vi "Obtain Message Queue.vi"(8 "error in (no error)":errorcluster) -> (0 "error out":errorcluster, 3 "Message Queue":refnum<queue>)   [LabVIEW 2020, in "Polar Bear Plus All-in-One Plugin.lvlib" / "Message Queue.lvlib"]
doc: "Create a queue with the Message Cluster data type."
uses:
  Message Queue.lvlib
  Message Cluster.ctl
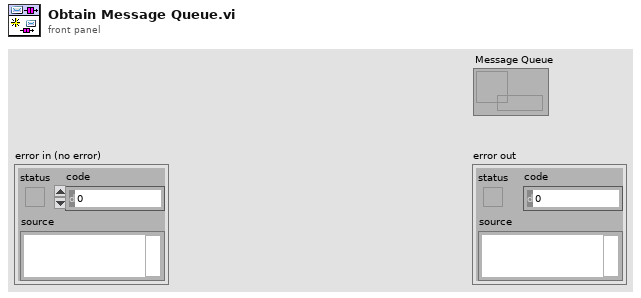
[diagram p1: front panel]
types:
  T1 = typedef "Polar Bear Plus All-in-One Plugin.lvlib/Message Queue.lvlib/Message Cluster.ctl" = cluster{"Message":string, "Message Data":variant}
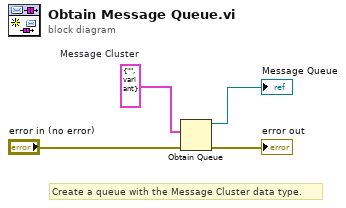
[diagram p0: block diagram]
diagram:
  w4 = T1 {"Message"="", "Message Data"=variant}  # Message Cluster
  # "Create a queue with the Message Cluster data type."
  n1 = Obtain Queue(element data type=w4, error in (no error)="error in (no error)") -> (queue out=→"Message Queue":refnum<queue>, error out=→"error out":errorcluster)  [unwired: 3 in, 1 out]
